vi "Open Database.vi"(6 "Standalone?":bool, 8 "error in (no error)":errorcluster, 11 "?":T1={"Server"="127.0.0.1", "Port"=3306, "UserID"="", "Password"="", "Database"=""}) -> (0 "error out":errorcluster, 3 ".Net dbase ref":refnum<k24>)   [LabVIEW 2017, in "VIs to Interface LabVIEW and MySQL dotNET Connector.lvlib"]
doc: "Use this VI to open a reference to a database using MySQL .NET Connector.\nIf Standalone? is True, the reference is closed at the end of execution - useful connection testing."
uses:
  VIs to Interface LabVIEW and MySQL dotNET Connector.lvlib
  MySql.Data
  Controls/Database Connection Data.ctl
panel:
  out "resulting string":string
  # "Use this VI to open a reference to a database using MySQL .NET Connector.\nIf Standalone? is True, the reference is closed at the end of execution - useful\nfor connection testing."
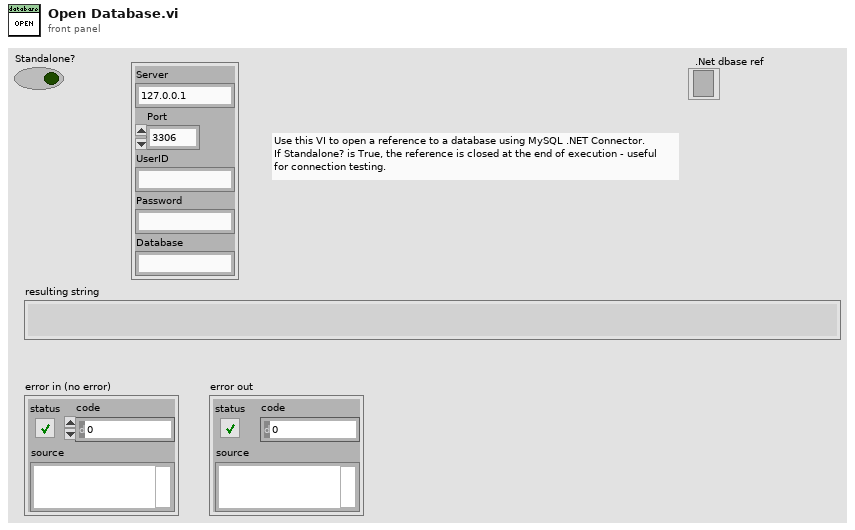
[diagram p1: front panel]
types:
  T1 = typedef "VIs to Interface LabVIEW and MySQL dotNET Connector.lvlib/Database Connection Data.ctl" = cluster{"Server":string, "Port":u32, "UserID":string, "Password":string, "Database":string}
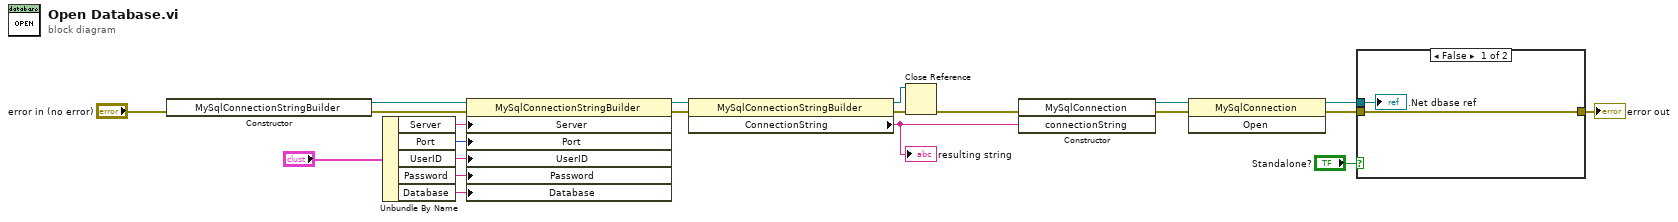
[diagram p0: block diagram]
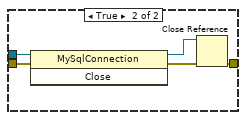
[diagram p2: hidden frame]
diagram:
  n1 = constructor class="MySqlConnectionStringBuilder"(error in="error in (no error)") -> (reference out=w14:refnum<k24>, error out=w13:errorcluster)  [unwired: 2 in, 1 out]
  n2 = Unbundle By Name("?") -> ("Server"=w5:string, "Port"=w4:u32, "UserID"=w3:string, "Password"=w2:string, "Database"=w1:string)
  n3 = property class="MySqlConnectionStringBuilder"(reference=w14, error in=w13, "Server"=w5, "Port"=w4, "UserID"=w3, "Password"=w2, "Database"=w1) -> (reference out=w17:refnum<k24>, error out=w21:errorcluster)
  n4 = property class="MySqlConnectionStringBuilder"(reference=w17, error in=w21) -> (reference out=w19:refnum<k24>, error out=w20:errorcluster, "ConnectionString"=w11:string)
  "resulting string" <- w11
  n5 = Close Reference(reference=w19, error in (no error)=w20) -> (error out=w10:errorcluster)
  n6 = constructor class="MySqlConnection"(error in=w10, "connectionString"=w11) -> (reference out=w8:refnum<k24>, error out=w9:errorcluster)  [unwired: 2 in, 2 out]
  n7 = invoke class="MySqlConnection" method="Open"(reference=w8, error in=w9) -> (reference out=w16:refnum<k24>, error out=w15:errorcluster)  [unwired: 1 in, 1 out]
  n8 = case shown="False" "Standalone?" {
    tunnel: [w23 w27] -> w18
    tunnel: w16 -> [w22 w25]
    tunnel: w15 -> [w23 w24]
    frame False {
      ".Net dbase ref" <- w22
    }
    frame True {
      n9 = invoke class="MySqlConnection" method="Close"(reference=w25, error in=w24) -> (reference out=w26:refnum<k24>, error out=w28:errorcluster)  [unwired: 1 in, 1 out]
      n10 = Close Reference(reference=w26, error in (no error)=w28) -> (error out=w27:errorcluster)
    }
  }
  "error out" <- w18
